vi "Problem 10 - Summation of primes.vi"() -> (3 "Answer":u64)   [LabVIEW 2021, in "Project Euler.lvlib"]
uses:
  Project Euler.lvlib
  Utilities/Named Timers/Named Timers.lvlib
  Utilities/Numeric Utilities/Numeric Utilities.lvlib
panel:
  out "Number of primes":i32
  out "Execution time (ms)":u32
  # "Development\nControls or indicators that are useful for development or testing, but which are not outputs of the VI."
  # "Input\nInputs to the VI"
  # "Output\nOutputs of the VI"
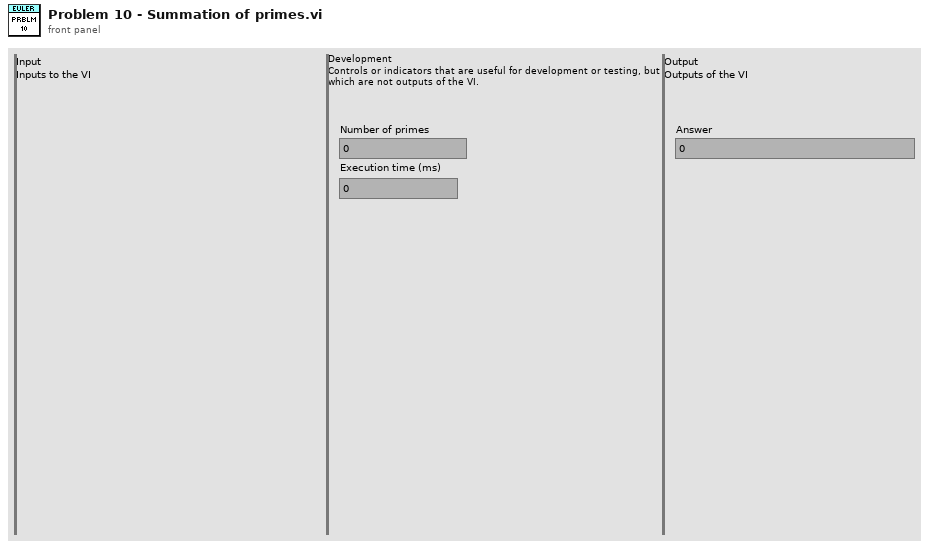
[diagram p1: front panel]
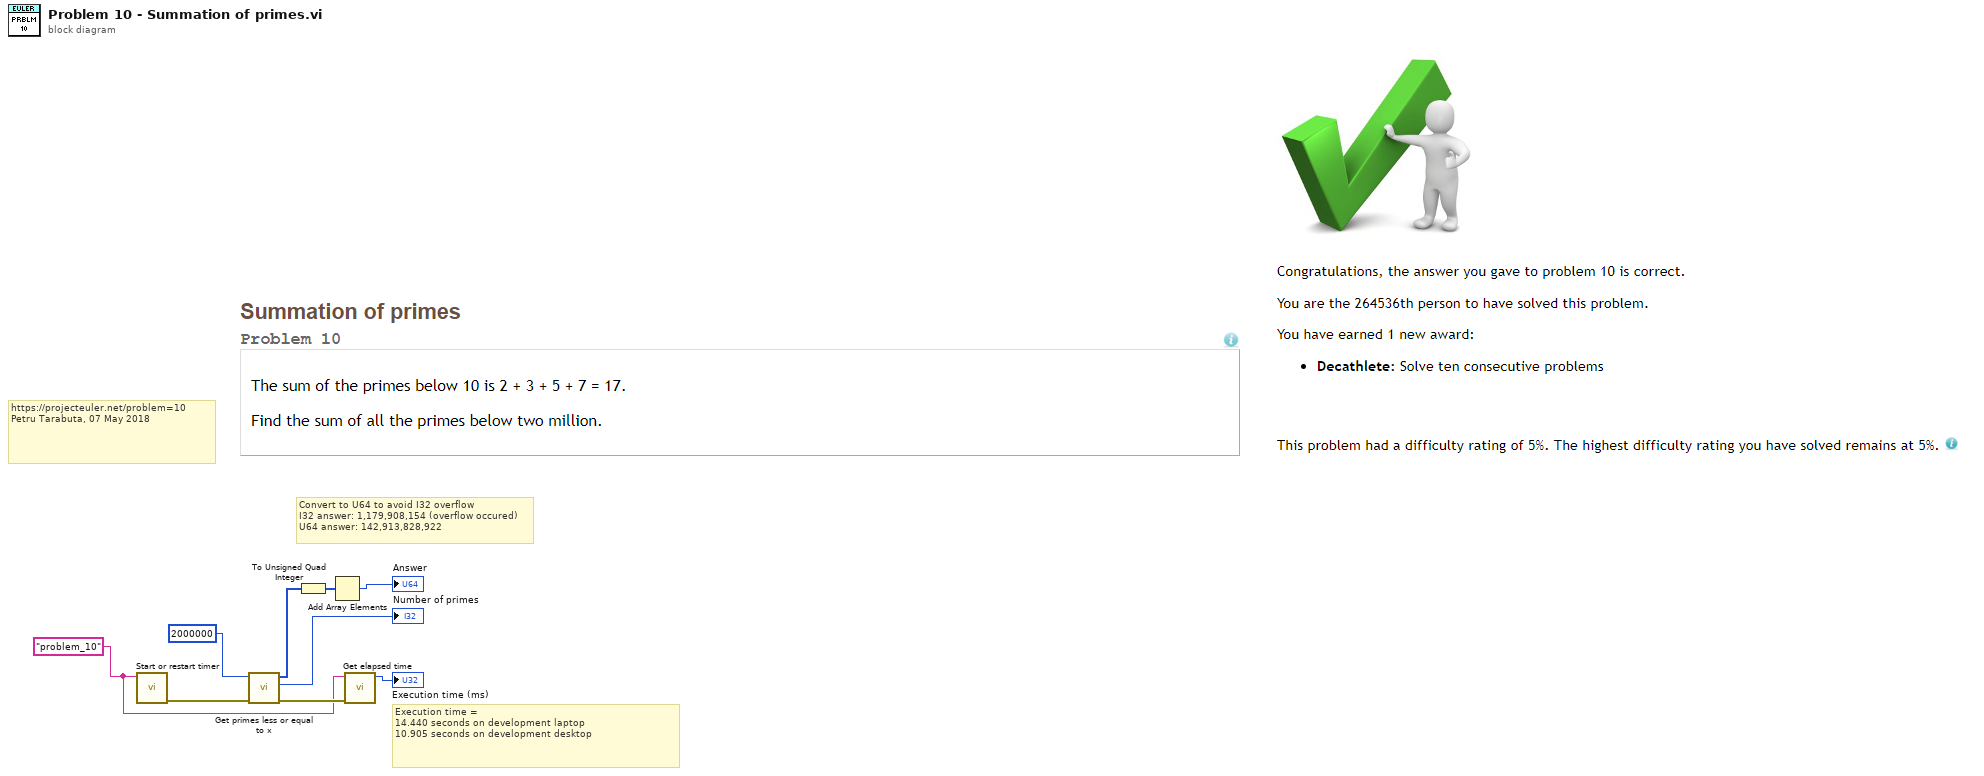
[diagram p0: block diagram]
diagram:
  w4 = "problem_10" ("Counter name (dflt=blank)")
  # "Convert to U64 to avoid I32 overflow\nI32 answer: 1,179,908,154 (overflow occured)\nU64 answer: 142,913,828,922"
  # "Execution time = \n14.440 seconds on development laptop\n10.905 seconds on development desktop"
  # "https://projecteuler.net/problem=10\nPetru Tarabuta, 07 May 2018"
  n1 = call "Start or restart timer.vi"("Timer name"=w4) -> ("error out"=w8:errorcluster)  [unwired: 10 in]
  n2 = call "Get primes less or equal to x.vi"("error in (no error)"=w8, "x = end"=2000000) -> ("error out"=w5:errorcluster, "Number of primes"=→"Number of primes":i32, "Primes"=w7:i32[])  [unwired: 7 in]
  n3 = To Unsigned Quad Integer(1:w7) -> (0:w1:u64[])
  n4 = Add Array Elements(numeric array=w1) -> (sum=→"Answer":u64)
  n5 = call "Get elapsed time.vi"("error in (no error)"=w5, "Timer name"=w4) -> ("Elapsed time (ms)"=→"Execution time (ms)":u32)  [unwired: 6 in, 3 out]
